vi "DAQdevice.vi"(11 "data in":dbl) -> (3 "data out":dynamicdata(waveform))   [LabVIEW 2025]
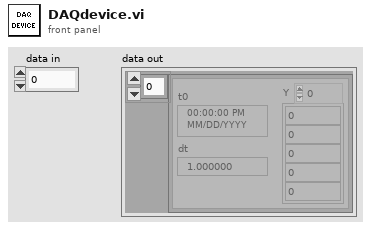
[diagram p1: front panel]
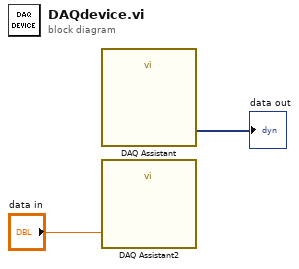
[diagram p0: block diagram]
diagram:
  n1 = call "DAQ Assistant"() -> ("data"=→"data out":dynamicdata)  [unwired: 17 in, 2 out]
  n2 = call "DAQ Assistant2"("data"="data in") -> ()  [unwired: 17 in, 2 out]
